vi "Pockels Cal-Display message gen.vi"(5 "Number of outer loop iteratons":i32=3, 7 "Index of current outer loop iteraton":i32=2, 8 "Pockels control voltage":dbl=-0.8 format="%#_gV", 9 "Index of current voltage step":i32=15, 10 "Number of voltage steps per objective":i32=21, 11 "Objective name string":string="Objective Name") -> (0 "error out":errorcluster)   [LabVIEW 2013]
uses:
  Globals/gl_Calibration globals.vi
panel:
  out "Progress %":u8=255
  out "Display Message":string
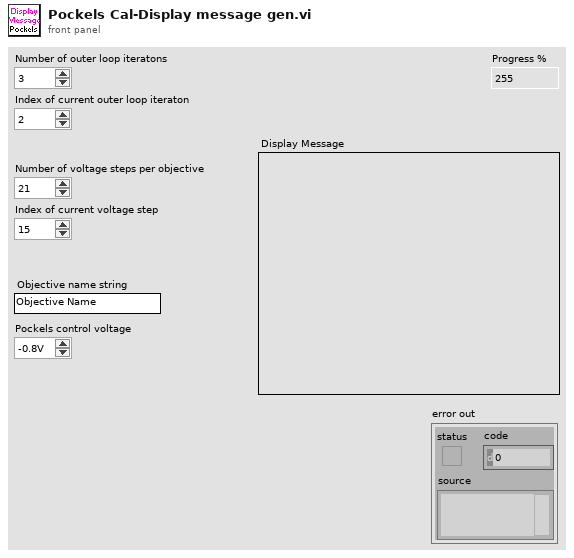
[diagram p1: front panel]
types:
  T1 = typedef "Cal mode.ctl" = enum16{"Automatic", "Interactive"}
  T2 = typedef "Pockels cal process refs.ctl" = cluster{"This VI":refnum<vi>, "Abort (ind)":refnum<vi>, "Next (ind)":refnum<vi>, "Cancel":refnum<vi>, "Next":refnum<vi>, "Message":refnum<vi>, "Measured Power ctrl":refnum<vi>, "Measured Power ind":refnum<vi>, "Pockels cal progress bar":refnum<vi>, "Abort this objective":refnum<vi>}
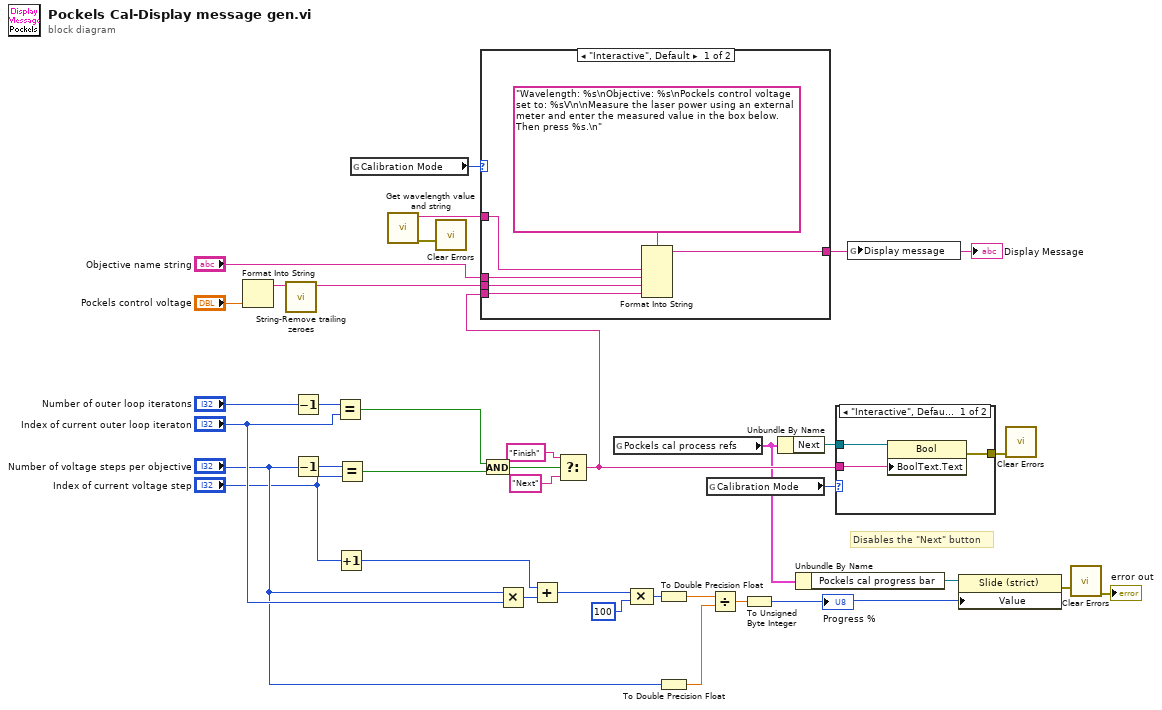
[diagram p0: block diagram]
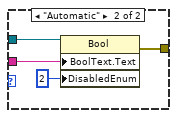
[diagram p2: hidden frame]
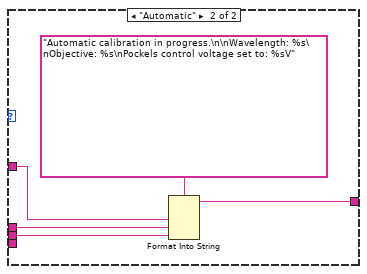
[diagram p3: hidden frame]
diagram:
  # "Disables the \"Next\" button"
  n1 = Format Into String("Pockels control voltage") -> (resulting string=w32:string)  [unwired: 3 in, 1 out]
  n2 = call "String-Remove trailing zeroes.vi"("String in"=w32) -> ("String out"=w11:string)  [unwired: 10 in]
  n3 = Decrement(x="Number of outer loop iteratons") -> (x-1=w28:i32)
  n4 = Decrement(x="Number of voltage steps per objective") -> (x-1=w27:i32)
  n5 = Equal?(x=w28, y="Index of current outer loop iteraton") -> (x = y?=w26:bool)
  n6 = Increment(x="Index of current voltage step") -> (x+1=w12:i32)
  n7 = Equal?(x=w27, y="Index of current voltage step") -> (x = y?=w18:bool)
  n8 = global read "gl_Calibration globals.vi" "Calibration Mode"() -> (w30:T1)
  n9 = call "Get wavelength value and string.vi"() -> ("error out"=w1:errorcluster, "Wavelength value string"=w7:string)  [unwired: 9 in, 1 out]
  n10 = call <vilib>:"Clear Errors.vi"("error in (no error)"=w1) -> ()  [unwired: 6 in, 1 out]
  n11 = And(x=w26, y=w18) -> (x .and. y?=w34:bool)
  n12 = Multiply(x="Number of voltage steps per objective", y="Index of current outer loop iteraton") -> (x*y=w14:i32)
  n13 = Add(x=w12, y=w14) -> (x+y=w15:i32)
  n14 = Select(t="Finish" ("Boolean Text.Text"), s=w34, f="Next" ("Boolean Text.Text")) -> (s? t:f=w10:string)
  n15 = case shown="\"Interactive\", Default" w30 {
    tunnel: "Objective name string" -> [w38 w44]
    tunnel: w11 -> [w42 w46]
    tunnel: [w39 w45] -> w9
    tunnel: w10 -> [w41 _]
    tunnel: w7 -> [w37 w43]
    frame "Interactive", Default {
      n16 = Format Into String(format string="Wavelength: %s\nObjective: %s\nPockels control voltage set to: %sV\n\nMeasure the laser power using an external meter and enter the measured value in the box below. Then press %s.\n", w37, w38, w42, w41) -> (resulting string=w39:string)  [unwired: 2 in, 1 out]
    }
    frame "Automatic" {
      n17 = Format Into String(format string="Automatic calibration in progress.\n\nWavelength: %s\nObjective: %s\nPockels control voltage set to: %sV", w43, w44, w46) -> (resulting string=w45:string)  [unwired: 2 in, 1 out]
    }
  }
  "Display Message" <- w9
  n18 = global read "gl_Calibration globals.vi" "Pockels cal process refs"() -> (w6:T2)
  n19 = Compound Arithmetic op=MULTIPLY(w15, 100 ("value")) -> (w23:i32)
  n20 = To Double Precision Float(number=w23) -> (double precision float=w22:dbl)
  n21 = To Double Precision Float(number="Number of voltage steps per objective") -> (double precision float=w21:dbl)
  n22 = global read "gl_Calibration globals.vi" "Calibration Mode"() -> (w29:T1)
  n23 = Divide(x=w22, y=w21) -> (x/y=w20:dbl)
  n24 = To Unsigned Byte Integer(number=w20) -> (unsigned 8bit integer=w4:u8)
  "Progress %" <- w4
  n25 = Unbundle By Name(w6) -> ("Next"=w31:refnum<vi>)
  n26 = Unbundle By Name(w6) -> ("Pockels cal progress bar"=w5:refnum<vi>)
  n27 = case shown="\"Interactive\", Default" w29 {
    tunnel: w31 -> [w50 w54]
    tunnel: w10 -> [w49 w53]
    tunnel: [w48 w51] -> w19
    frame "Interactive", Default {
      n28 = property on="Property Node" class="Bool"(reference=w50, "BoolText.Text"=w49) -> (error out=w48:errorcluster)  [unwired: 1 in, 1 out]
    }
    frame "Automatic" {
      n29 = property on="Property Node" class="Bool"(reference=w54, "BoolText.Text"=w53, "DisabledEnum"=2) -> (error out=w51:errorcluster)  [unwired: 1 in, 1 out]
    }
  }
  n30 = global write "gl_Calibration globals.vi" "Display message"(w9) -> ()
  n31 = property class="Slide (strict)"(reference=w5, "Value"=w4) -> (error out=w3:errorcluster)  [unwired: 1 in, 1 out]
  n32 = call <vilib>:"Clear Errors.vi"("error in (no error)"=w19) -> ()  [unwired: 6 in, 1 out]
  n33 = call <vilib>:"Clear Errors.vi"("error in (no error)"=w3) -> ("error out"=→"error out":errorcluster)  [unwired: 6 in]
